vi "GSP_Manager_CF.vi"() -> ()   [LabVIEW 2015]
uses:
  SystemUtil/ScriptArray.ctl
  SystemUtil/Script.ctl
  SystemUtil/Command.ctl
  SystemUtil/MotorStates.ctl
  piezo_setpoint.ctl
  SystemUtil/ThreadStates.ctl
  Log/LogItem.ctl
  GSP_CF_Global.vi
  GUI/GSP_GUI_global.vi
panel:
  in  "Change CF":bool
  in  "CF Target":i32 caption="Target" min=-3000 max=3000
  out "CF Actual":i32 caption="Actual"
  out "Cameral Ext Temp":dbl(slide) scale=0.0..20.0
  out "Last Error":errorcluster
  in  "CommandQ":string
  # "Camera Focus"
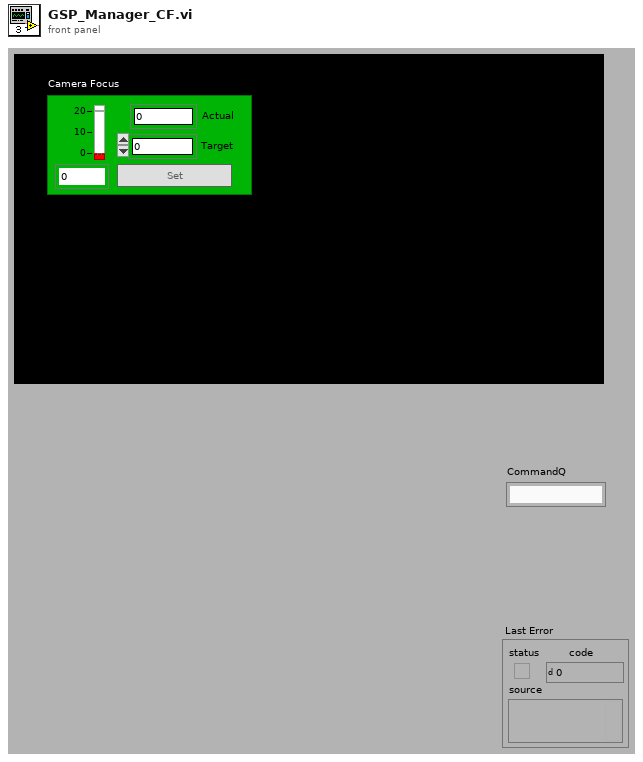
[diagram p1: front panel]
types:
  T1 = typedef "Command.ctl" = cluster{"Command":string, "Parameter":string}
  T2 = typedef "ScriptArray.ctl" = T3[]
  T3 = typedef "Script.ctl" = cluster{"Current Step":i32, "Commands":cluster{"Command":string, "Parameters":string}[]}
  T4 = cluster{"Move Mem Address":i32, "Home Mem Address":i32, "Adjust Piezo Address":i32}
  T5 = typedef "MotorStates.ctl" = enum16{"Ready", "Moving", "Uninitialized", "Error"}
  T6 = typedef "piezo_setpoint.ctl" = cluster{"Left":i32, "Right":i32}
  T7 = typedef "ThreadStates.ctl" = enum16{"Waiting", "Scripting", "Uninitialized", "Error"}
  T8 = enum16{"Launch", "Log", "Open", "Close", "Shutdown"}
  T9 = typedef "LogItem.ctl" = cluster{"error in (no error)":errorcluster, "Source":string, "Comment ":string}
  T10 = enum16{"POL (0)", "CPL (1)", "HLT (2)", "STP (3)", "RST (4)", "RVN (5)", "RPB (6)", "CLP (8)", "SDL (9)", "RUN (10)", "WRI (11)", "RRG (12)", "SPR (13)", "LPR (14)", "VMI (15)", "SSP (17)", "SSE (18)", "RIS (20)", "RIO (21)", "IMW (25)", "END (128)", "MAV (134)", "MRV (135)", "JRE (137)", "WCL (138)", "WCW (139)", "DLY (140)", "WDL (141)", "GCL (142)", "GOP (143)", "ZTG (144)", "ZTP (145)", "TTP (146)", "CME (147)", "CTC (148)", "TQL (149)", "AHC (150)", "ERL (151)", "OLP (152)", "WRP (154)", "IDT (155)", "LRP (156)", "VMP (159)", "RAV (160)", "RRV (161)", "JMP (162)", "JOI (162)", "CIS (163)", "CKS (164)", "CLC (165)", "KMC (167)", "MCT (168)", "FLC (169)", "EEM (170)", "DDB (171)", "DEM (171)", "PAC (172)", "ADL (173)", "BRT (174)", "MAT (176)", "MRT (177)", "RAT (178)", "RRT (179)", "SSD (180)", "KMR (181)", "KED (182)", "KDD (183)", "DIR (184)", "PRO (185)", "SIF (186)", "EDL (187)", "CIO (188)", "MDS (189)", "MDC (190)", "MDT (191)", "SEE (192)", "ARI (193)", "WBS (194)", "SCF (195)", "RSM (196)", "RLM (197)", "RSN (198)", "RLN (199)", "PCL (201)", "PCI (201)", "PRT (202)", "PRI (202)", "WBE (204)", "SOB (205)", "COB (206)", "ACR (207)", "PLR (208)", "CAI (211)", "LVT (212)", "OVT (213)", "MTT (214)", "CLC (215)", "PIM (216)", "VIM (217)", "TIM (218)", "AHM (219)", "SSL (221)", "TRU (222)", "RSD (223)", "EMT (225)", "DMT (226)", "EMD (227)", "DMD (228)", "HSM (229)", "AHD (230)", "PCM (231)", "PCG (232)", "XRV (233)", "XAV (234)", "XRT (235)", "XAT (236)", "GOC (237)", "JNA (238)", "JOR (239)", "PMC (240)", "PMV (241)", "PMX (242)", "DLC (243)", "SLC (244)", "PCP (245)", "ATR (248)", "PMO (249)", "JAN (250)", "EDH (251)", "DIF (252)", "IMS (253)", "IMQ (254)"}
  T11 = cluster{"Mount Az":dbl, "Mount El":dbl, "RA":string, "DEC":string, "Hour Angle":string, "Airmass":dbl, "Focus":dbl, "Rotator Angle":dbl, "Rotator Location":string, "Dome Shutter":string, "Dome Az":dbl, "Date":string, "UT Time":string, "Sidereal Time":string, "Position Angle":dbl, "Seeing":dbl, "OBSRA":string, "OBSDEC":string, "Position ADC":string, "Position ADC 2":string}
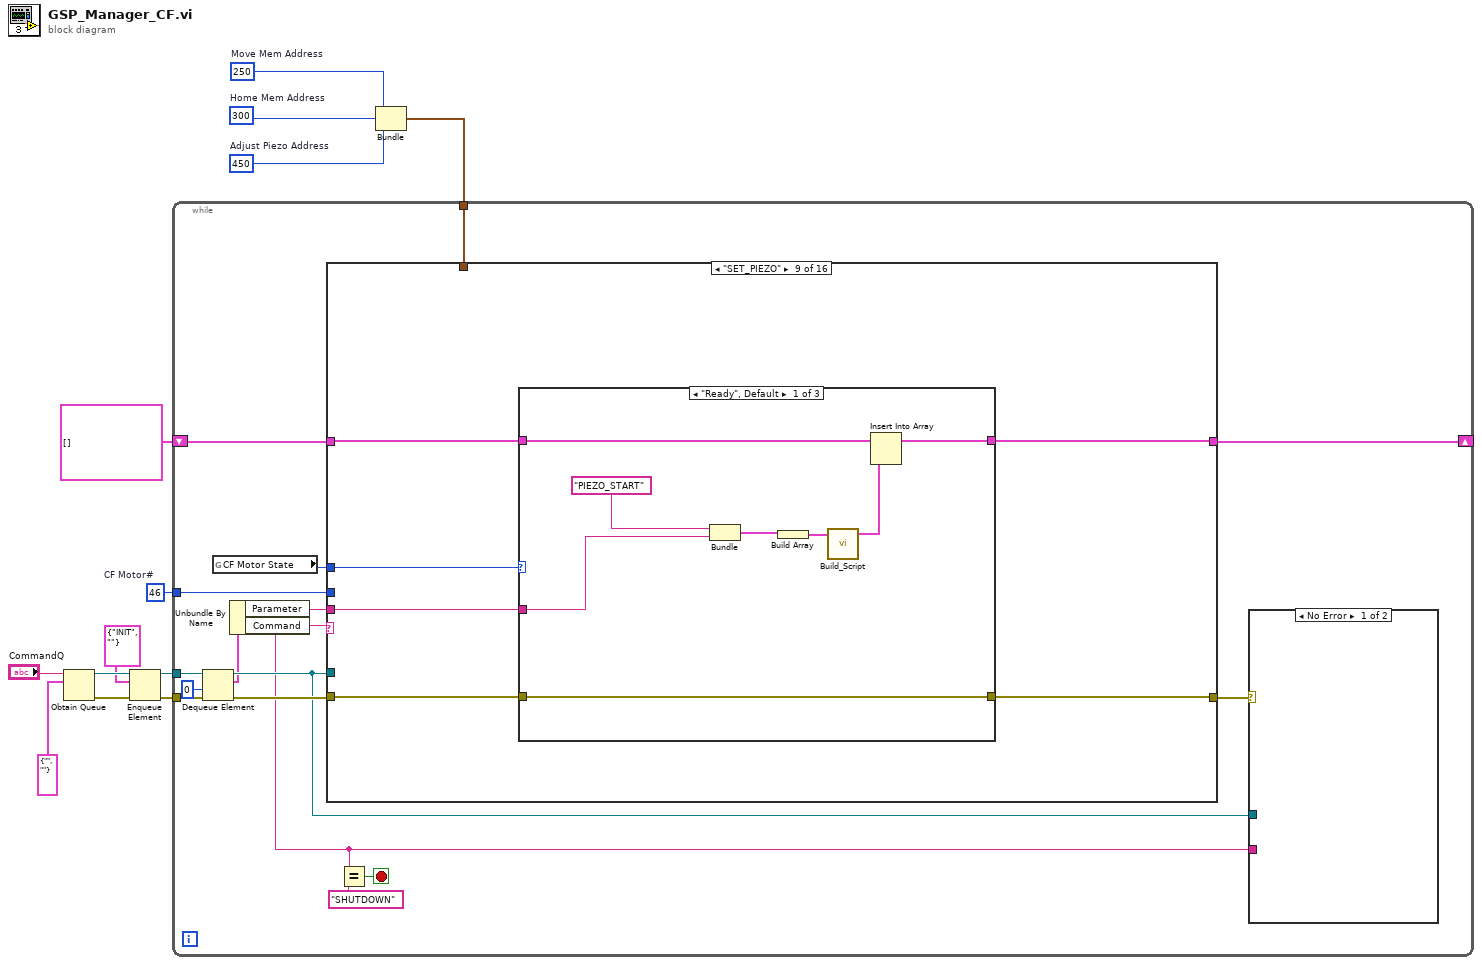
[diagram p0: block diagram]
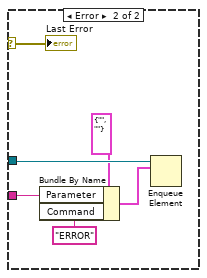
[diagram p2: hidden frame]
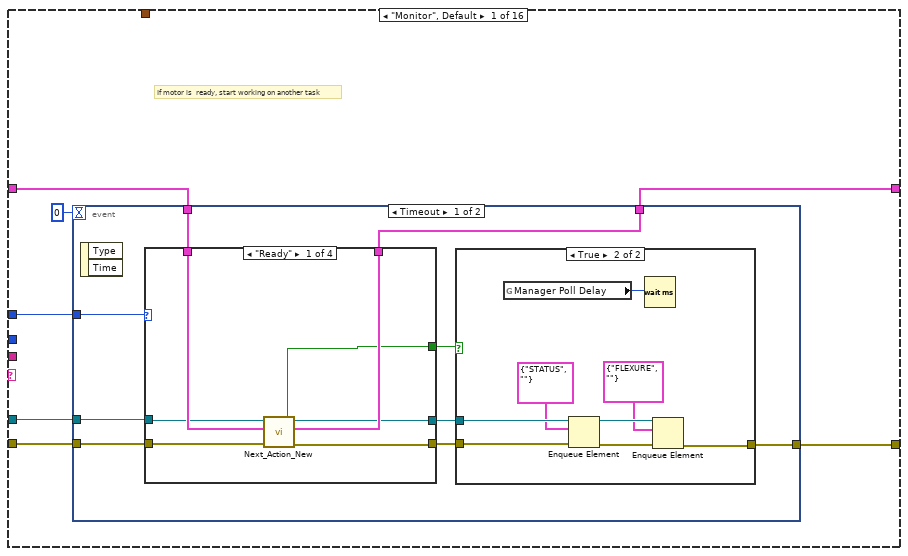
[diagram p3: hidden frame]
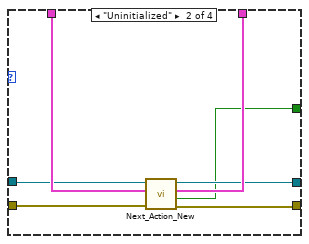
[diagram p5: hidden frame]
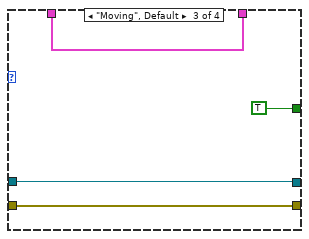
[diagram p6: hidden frame]
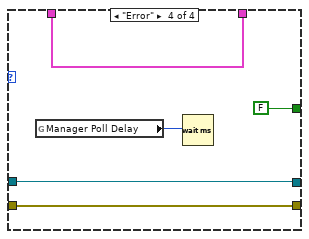
[diagram p7: hidden frame]
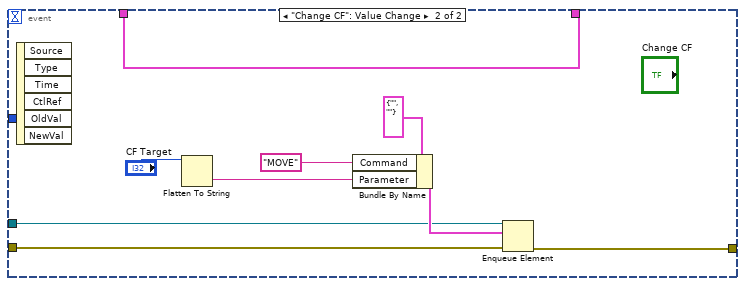
[diagram p8: hidden frame]
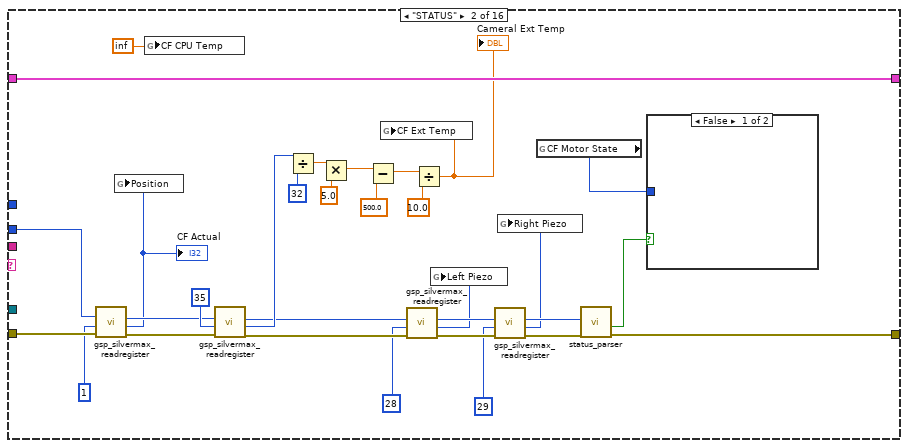
[diagram p9: hidden frame]
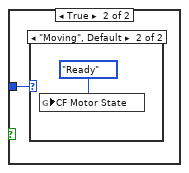
[diagram p10: hidden frame]
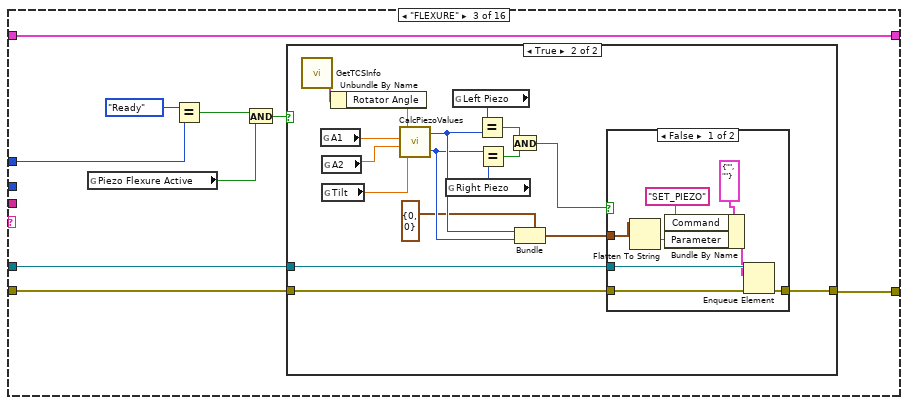
[diagram p12: hidden frame]
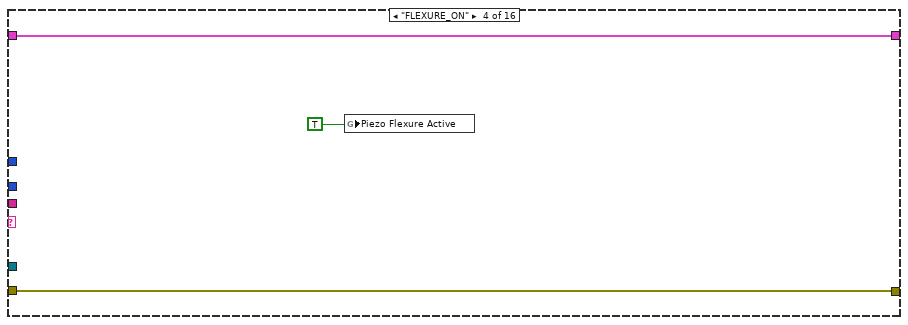
[diagram p15: hidden frame]
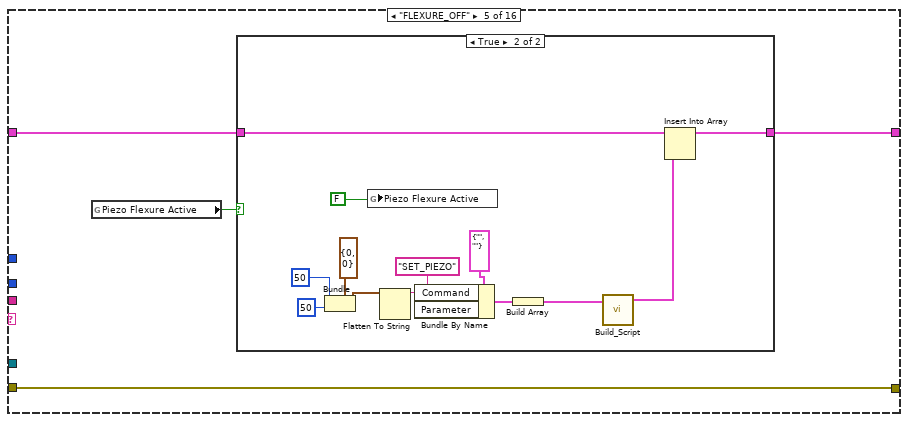
[diagram p16: hidden frame]
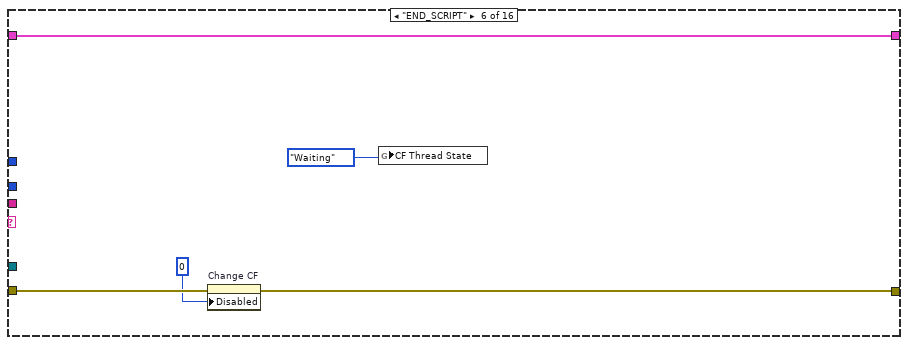
[diagram p18: hidden frame]
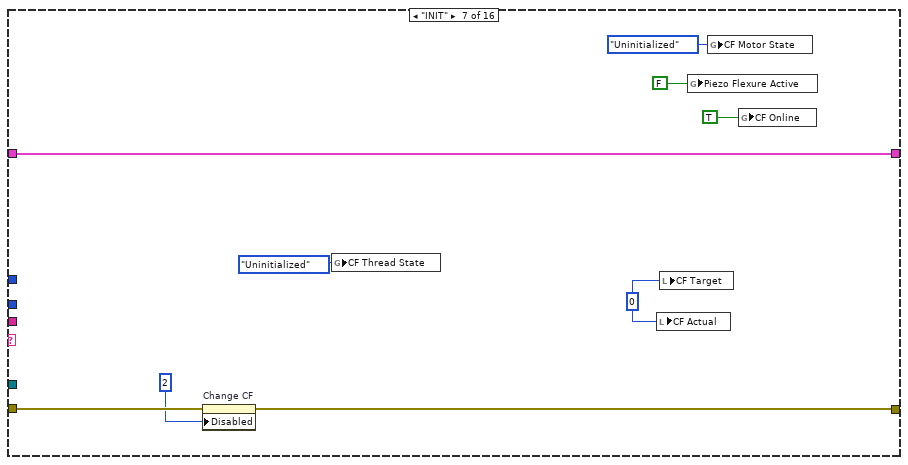
[diagram p19: hidden frame]
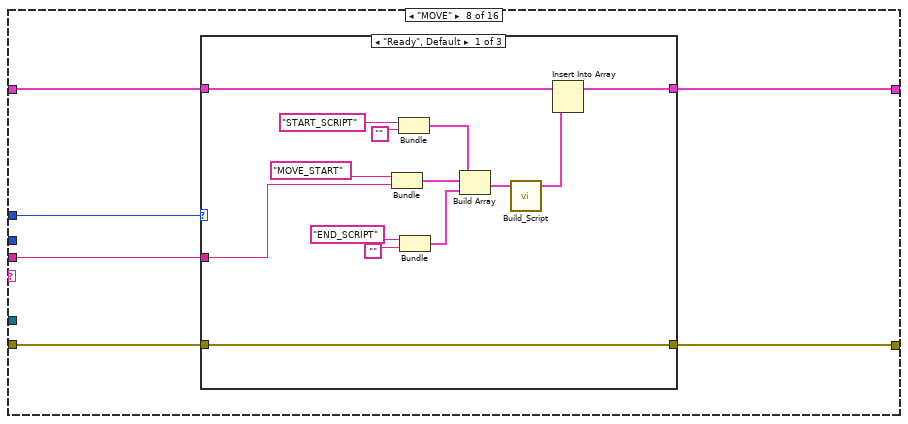
[diagram p20: hidden frame]
diagram:
  w1 = 450  # Adjust Piezo Address
  w3 = 300  # Home Mem Address
  w4 = 250  # Move Mem Address
  w5 = u8 46  # CF Motor#
  n1 = Obtain Queue(name (unnamed)="CommandQ", element data type=T1 {"Command"="", "Parameter"=""} ("Command")) -> (queue out=w10:refnum<queue>, error out=w11:errorcluster)  [unwired: 3 in, 1 out]
  n2 = Enqueue Element(queue=w10, element=T1 {"Command"="INIT", "Parameter"=""}, error in (no error)=w11) -> (queue out=w13:refnum<queue>, error out=w12:errorcluster)  [unwired: 1 in, 1 out]
  n3 = Bundle("Move Mem Address"=w4, "Home Mem Address"=w3, "Adjust Piezo Address"=w1) -> (w2:T4)  [unwired: 1 in]
  n4 = while {
    tunnel: w13 -> [w29]
    tunnel: w12 -> [w28]
    tunnel: w5 -> [w23]
    shift-right: [w22] -> _
    shift-left: T2 [] ("Operations") -> [w21]
    tunnel: w2 -> [w14]
    stop <- w17 stop-if-true
    n5 = Dequeue Element(queue=w29, timeout in ms (-1)=0, error in (no error)=w28) -> (queue out=w25:refnum<queue>, element=w19:T1, error out=w27:errorcluster)  [unwired: 1 out]
    n6 = global read "GSP_CF_Global.vi" "CF Motor State"() -> (w15:T5)
    n7 = Unbundle By Name(w19) -> ("Parameter"=w18:string, "Command"=w16:string)
    n8 = case shown="\"SET_PIEZO\"" w16 {
      tunnel: w27 -> [w41 w123 w131 w162 w166 w184 w189 w199 w235 w263 w282 w310 w316 w321 w324 _]
      tunnel: w25 -> [w42 _ w130 _ _ _ _ _ _ _ _ w311 _ _ _ w344]
      tunnel: [w37 w120 w129 w162 w166 w185 w190 w198 w234 w273 w298 w309 w314 w321 w330 _] -> w26
      tunnel: w23 -> [_ w122 _ _ _ _ _ _ _ w267 w290 _ _ _ w333 _]
      tunnel: w21 -> [w40 w118 w134 w164 w168 w187 w195 w202 w238 w270 w295 w312 w318 w323 w327 w338]
      tunnel: [w39 w118 w134 w164 w167 w187 w195 w201 w237 w270 w295 w312 w318 w322 w327 w337] -> w22
      tunnel: w18 -> [_ _ _ _ _ _ _ w200 w236 w268 w294 _ _ _ _ _]
      tunnel: w15 -> [w38 _ w127 _ _ _ _ w197 w233 _ _ _ _ _ _ _]
      tunnel: w14 -> [_ _ _ _ _ _ _ _ _ w266 w284 _ _ _ w326 _]
      frame "Monitor", Default {
        # "If motor is  ready, start working on another task"
        n9 = event shown="[0] Timeout" {
          selector: _ -> [_ _]
          dyn-events: _ -> [_ _]
          timeout: 0 -> [_ _]
          tunnel: w42 -> [w51 w88]
          tunnel: w41 -> [w50 w87]
          tunnel: w40 -> [w49 w84]
          tunnel: [w48 w84] -> w39
          tunnel: w38 -> [w47 _]
          tunnel: [w43 w86] -> w37
          event Timeout {
            n10 = event-data() -> ()  [unwired: 1 in, 2 out]
            n11 = case shown="\"Ready\"" w47 {
              tunnel: w51 -> [w63 w70 w77 w80]
              tunnel: w50 -> [w67 w74 w76 w82]
              tunnel: [w65 w72 w76 w82] -> w46
              tunnel: w49 -> [w66 w73 w78 w83]
              tunnel: [w64 w71 w78 w83] -> w48
              tunnel: [w62 w68 TRUE FALSE] -> w45
              tunnel: [w61 w69 w77 w80] -> w44
              frame "Ready" {
                n12 = call "Next_Action_New.vi"("error in (no error)"=w67, "Operations"=w66, "queue in"=w63) -> ("error out"=w65:errorcluster, "No command?"=w62:bool, "Operations Out"=w64:T2, "queue out"=w61:refnum<queue>)  [unwired: 1 in]
              }
              frame "Uninitialized" {
                n13 = call "Next_Action_New.vi"("error in (no error)"=w74, "Operations"=w73, "queue in"=w70) -> ("error out"=w72:errorcluster, "No command?"=w68:bool, "Operations Out"=w71:T2, "queue out"=w69:refnum<queue>)  [unwired: 1 in]
              }
              frame "Moving", Default {
              }
              frame "Error" {
                n14 = global read "GSP_GUI_global.vi" "Manager Poll Delay"() -> (w81:u32)
                n15 = Wait (ms)(milliseconds to wait=w81) -> ()  [unwired: 1 out]
              }
            }
            n16 = case shown="True" w45 {
              tunnel: w46 -> [w52 w60]
              tunnel: w44 -> [_ w59]
              tunnel: [w52 w53] -> w43
              frame False {
              }
              frame True {
                n17 = global read "GSP_GUI_global.vi" "Manager Poll Delay"() -> (w58:u32)
                n18 = Enqueue Element(queue=w59, element=T1 {"Command"="STATUS", "Parameter"=""}, error in (no error)=w60) -> (queue out=w57:refnum<queue>, error out=w56:errorcluster)  [unwired: 1 in, 1 out]
                n19 = Wait (ms)(milliseconds to wait=w58) -> ()  [unwired: 1 out]
                n20 = Enqueue Element(queue=w57, element=cluster{"Command":string, "Parameters":string} {"Command"="FLEXURE", "Parameters"=""} ("Default Command"), error in (no error)=w56) -> (error out=w53:errorcluster)  [unwired: 1 in, 2 out]
              }
            }
          }
          event "Change CF": Value Change {
            n21 = event-data() -> ()  [unwired: 1 in, 6 out]
            n22 = Flatten To String(anything="CF Target") -> (data string=w89:string)  [unwired: 3 in, 2 out]
            n23 = Bundle By Name(cluster=T1 {"Command"="", "Parameter"=""} ("element"), "Command"="MOVE" ("element"), "Parameter"=w89) -> (w91:T1)
            n24 = Enqueue Element(queue=w88, element=w91, error in (no error)=w87) -> (error out=w86:errorcluster)  [unwired: 1 in, 2 out]
          }
        }
      }
      frame "STATUS" {
        n25 = call "gsp_silvermax_readregister.vi"("error in (no error)"=w123, "Register# (0)"=u8 1, "Motor #"=w122) -> ("error out"=w115:errorcluster, "Register Value"=w93:i32, "Motor # dup"=w116:u8)  [unwired: 2 in, 2 out]
        "CF Actual" <- w93
        n26 = global write "GSP_CF_Global.vi" "Position"(w93) -> ()
        n27 = global write "GSP_CF_Global.vi" "CF CPU Temp"(inf) -> ()
        n28 = call "gsp_silvermax_readregister.vi"("error in (no error)"=w115, "Register# (0)"=u8 35, "Motor #"=w116) -> ("error out"=w105:errorcluster, "Register Value"=w106:i32, "Motor # dup"=w104:u8)  [unwired: 2 in, 2 out]
        n29 = Divide(x=w106, y=32) -> (x/y=w113:dbl)
        n30 = Multiply(x=w113, y=5.0) -> (x*y=w111:dbl)
        n31 = Subtract(x=w111, y=500.0) -> (x-y=w109:dbl)
        n32 = call "gsp_silvermax_readregister.vi"("error in (no error)"=w105, "Register# (0)"=u8 28, "Motor #"=w104) -> ("error out"=w102:errorcluster, "Register Value"=w97:i32, "Motor # dup"=w100:u8)  [unwired: 2 in, 2 out]
        n33 = Divide(x=w109, y=10.0) -> (x/y=w94:dbl)
        "Cameral Ext Temp" <- w94
        n34 = global write "GSP_CF_Global.vi" "CF Ext Temp"(w94) -> ()
        n35 = global write "GSP_CF_Global.vi" "Left Piezo"(w97) -> ()
        n36 = call "gsp_silvermax_readregister.vi"("error in (no error)"=w102, "Register# (0)"=u8 29, "Motor #"=w100) -> ("error out"=w101:errorcluster, "Register Value"=w96:i32, "Motor # dup"=w99:u8)  [unwired: 2 in, 2 out]
        n37 = global write "GSP_CF_Global.vi" "Right Piezo"(w96) -> ()
        n38 = global read "GSP_CF_Global.vi" "CF Motor State"() -> (w95:T5)
        n39 = call "status_parser.vi"("error in (no error)"=w101, "Motor #"=w99) -> ("error out"=w120:errorcluster, "Program Complete?"=w119:bool)  [unwired: 3 in, 1 out]
        n40 = case shown="False" w119 {
          tunnel: w95 -> [_ w124]
          frame False {
          }
          frame True {
            n41 = case shown="\"Moving\", Default" w124 {
              frame "Uninitialized" {
              }
              frame "Moving", Default {
                n42 = global write "GSP_CF_Global.vi" "CF Motor State"(MotorStates."Ready" ("Mode")) -> ()
              }
            }
          }
        }
      }
      frame "FLEXURE" {
        n43 = global read "GSP_CF_Global.vi" "Piezo Flexure Active"() -> (w128:bool)
        n44 = Equal?(x=MotorStates."Ready", y=w127) -> (x = y?=w133:bool)
        n45 = And(x=w133, y=w128) -> (x .and. y?=w132:bool)
        n46 = case shown="True" w132 {
          tunnel: w131 -> [w135 w143]
          tunnel: w130 -> [_ w144]
          tunnel: [w135 w145] -> w129
          frame False {
          }
          frame True {
            n47 = call "GetTCSInfo.vi"() -> ("TCSInfo"=w137:T11)
            n48 = global read "GSP_CF_Global.vi" "A1"() -> (w152:dbl)
            n49 = global read "GSP_CF_Global.vi" "A2"() -> (w151:dbl)
            n50 = global read "GSP_CF_Global.vi" "Tilt"() -> (w150:dbl)
            n51 = Unbundle By Name(w137) -> ("Rotator Angle"=w136:dbl)
            n52 = call "CalcPiezoValues.vi"("Tilt"=w150, "A2"=w151, "A1"=w152, "Rotator Position"=w136) -> ("Right Piezo"=w141:i32, "Left Piezo"=w142:i32)
            n53 = global read "GSP_CF_Global.vi" "Right Piezo"() -> (w148:i32)
            n54 = global read "GSP_CF_Global.vi" "Left Piezo"() -> (w149:i32)
            n55 = Equal?(x=w149, y=w142) -> (x = y?=w147:bool)
            n56 = Equal?(x=w141, y=w148) -> (x = y?=w146:bool)
            n57 = And(x=w147, y=w146) -> (x .and. y?=w140:bool)
            n58 = Bundle(cluster=T6 {"Left"=0, "Right"=0} ("Piezos Setpoints"), "Left"=w142, "Right"=w141) -> (w139:T6)
            n59 = case shown="False" w140 {
              tunnel: [w160 w161] -> w145
              tunnel: w144 -> [w159 _]
              tunnel: w143 -> [w158 w161]
              tunnel: w139 -> [w154 _]
              frame False {
                n60 = Flatten To String(anything=w154) -> (data string=w153:string)  [unwired: 3 in, 2 out]
                n61 = Bundle By Name(cluster=T1 {"Command"="", "Parameter"=""} ("element"), "Command"="SET_PIEZO", "Parameter"=w153) -> (w155:T1)
                n62 = Enqueue Element(queue=w159, element=w155, error in (no error)=w158) -> (error out=w160:errorcluster)  [unwired: 1 in, 2 out]
              }
              frame True {
              }
            }
          }
        }
      }
      frame "FLEXURE_ON" {
        n63 = global write "GSP_CF_Global.vi" "Piezo Flexure Active"(TRUE) -> ()
      }
      frame "FLEXURE_OFF" {
        n64 = global read "GSP_CF_Global.vi" "Piezo Flexure Active"() -> (w165:bool)
        n65 = case shown="True" w165 {
          tunnel: w168 -> [w169 w174]
          tunnel: [w169 w170] -> w167
          frame False {
          }
          frame True {
            n66 = Bundle(cluster=T6 {"Left"=0, "Right"=0} ("Piezos Setpoints"), "Left"=50, "Right"=50) -> (w177:T6)
            n67 = global write "GSP_CF_Global.vi" "Piezo Flexure Active"(FALSE) -> ()
            n68 = Flatten To String(anything=w177) -> (data string=w179:string)  [unwired: 3 in, 2 out]
            n69 = Bundle By Name(cluster=T1 {"Command"="", "Parameter"=""} ("element"), "Command"="SET_PIEZO", "Parameter"=w179) -> (w172:T1)
            n70 = Build Array(w172) -> (w171:T1[])
            n71 = call "Build_Script.vi"("Commands"=w171) -> ("script out"=w173:T3)  [unwired: 4 in]
            n72 = Insert Into Array(array=w174, new element=w173) -> (w170:T2)  [unwired: 1 in]
          }
        }
      }
      frame "END_SCRIPT" {
        n73 = property on="Change CF" class="Bool"(error in=w184, "Disabled"=u8 0) -> (error out=w185:errorcluster)  [unwired: 1 in, 1 out]
        n74 = global write "GSP_CF_Global.vi" "CF Thread State"(ThreadStates."Waiting" ("Thread state")) -> ()
      }
      frame "INIT" {
        w191 = 0 ("Value")
        n75 = property on="Change CF" class="Bool"(error in=w189, "Disabled"=u8 2) -> (error out=w190:errorcluster)  [unwired: 1 in, 1 out]
        n76 = global write "GSP_CF_Global.vi" "CF Thread State"(ThreadStates."Uninitialized" ("Thread state")) -> ()
        n77 = local write "CF Actual"(w191) -> ()
        n78 = local write "CF Target"(w191) -> ()
        n79 = global write "GSP_CF_Global.vi" "Piezo Flexure Active"(FALSE) -> ()
        n80 = global write "GSP_CF_Global.vi" "CF Motor State"(MotorStates."Uninitialized" ("Mode")) -> ()
        n81 = global write "GSP_CF_Global.vi" "CF Online"(TRUE ("CS Online")) -> ()
      }
      frame "MOVE" {
        n82 = case shown="\"Ready\", Default" w197 {
          tunnel: w202 -> [w216 w218 w226]
          tunnel: [w215 w218 w226] -> w201
          tunnel: w200 -> [w209 _ _]
          tunnel: w199 -> [w214 w224 w232]
          tunnel: [w214 w223 w231] -> w198
          frame "Ready", Default {
            n83 = Bundle("MOVE_START", "Parameter"=w209) -> (w208:cluster{string, "Parameter":string})  [unwired: 1 in]
            n84 = Bundle("START_SCRIPT", "") -> (w203:cluster{string, string})  [unwired: 1 in]
            n85 = Bundle("END_SCRIPT", "") -> (w207:cluster{string, string})  [unwired: 1 in]
            n86 = Build Array(w203, w208, w207) -> (w206:cluster{string, "Parameter":string}[])
            n87 = call "Build_Script.vi"("Commands"=w206) -> ("script out"=w213:T3)  [unwired: 4 in]
            n88 = Insert Into Array(array=w216, new element=w213) -> (w215:T2)  [unwired: 1 in]
          }
          frame "Uninitialized" {
            n89 = Bundle By Name(cluster=T9 {"error in (no error)"={"status"=FALSE, "code"=0, "source"=""}, "Source"="", "Comment "=""} ("Log"), "Source"="Coll Focus Manager", "Comment"="Cannot perform move") -> (w222:T9)
            n90 = call "GSP_Logger_Handler.vi"("error in (no error)"=w224, "Log"=w222, "Actions"=T8."Log") -> ("error out"=w223:errorcluster)  [unwired: 4 in]
          }
          frame "Error" {
            n91 = Bundle By Name(cluster=T9 {"error in (no error)"={"status"=FALSE, "code"=0, "source"=""}, "Source"="", "Comment "=""} ("Log"), "Source"="Coll Focus Manager", "Comment"="Cannot perform move") -> (w230:T9)
            n92 = call "GSP_Logger_Handler.vi"("error in (no error)"=w232, "Log"=w230, "Actions"=T8."Log") -> ("error out"=w231:errorcluster)  [unwired: 4 in]
          }
        }
      }
      frame "SET_PIEZO" {
        n93 = case shown="\"Ready\", Default" w233 {
          tunnel: w238 -> [w246 w248 w256]
          tunnel: [w245 w248 w256] -> w237
          tunnel: w236 -> [w241 _ _]
          tunnel: w235 -> [w244 w254 w262]
          tunnel: [w244 w253 w261] -> w234
          frame "Ready", Default {
            n94 = Bundle("PIEZO_START", "Parameter"=w241) -> (w240:cluster{string, "Parameter":string})  [unwired: 1 in]
            n95 = Build Array(w240) -> (w239:cluster{string, "Parameter":string}[])
            n96 = call "Build_Script.vi"("Commands"=w239) -> ("script out"=w243:T3)  [unwired: 4 in]
            n97 = Insert Into Array(array=w246, new element=w243) -> (w245:T2)  [unwired: 1 in]
          }
          frame "Uninitialized" {
            n98 = Bundle By Name(cluster=T9 {"error in (no error)"={"status"=FALSE, "code"=0, "source"=""}, "Source"="", "Comment "=""} ("Log"), "Source"="Camera Focus Manager", "Comment"="Cannot perform move") -> (w252:T9)
            n99 = call "GSP_Logger_Handler.vi"("error in (no error)"=w254, "Log"=w252, "Actions"=T8."Log") -> ("error out"=w253:errorcluster)  [unwired: 4 in]
          }
          frame "Error" {
            n100 = Bundle By Name(cluster=T9 {"error in (no error)"={"status"=FALSE, "code"=0, "source"=""}, "Source"="", "Comment "=""} ("Log"), "Source"="Camera Focus Manager", "Comment"="Cannot perform move") -> (w260:T9)
            n101 = call "GSP_Logger_Handler.vi"("error in (no error)"=w262, "Log"=w260, "Actions"=T8."Log") -> ("error out"=w261:errorcluster)  [unwired: 4 in]
          }
        }
      }
      frame "MOVE_START" {
        n102 = Unflatten From String(type=0, binary string=w268) -> (value=w264:i32)  [unwired: 3 in, 2 out]
        n103 = Unbundle By Name(w266) -> ("Move Mem Address"=w265:i32)
        n104 = local write "CF Target"(w264) -> ()
        n105 = global write "GSP_CF_Global.vi" "Target"(w264) -> ()
        n106 = Number To Decimal String(number=w265) -> (decimal integer string=w272:string)  [unwired: 1 in]
        n107 = call "gsp_silvermax_writeregister.vi"("error in (no error)"=w263, "Register Value"=w264, "Motor #"=w267, "Register# (0)"=u8 25) -> ("error out"=w277:errorcluster, "Motor # dup"=w275:u8)  [unwired: 2 in]
        n108 = Build Array(w272) -> (w271:string[])
        n109 = call "gsp_silvermax_commandreponse.vi"("error in (no error)"=w277, "Parameters (none)"=w271, "Motor #"=w275, "Command"=T10."LRP (156)") -> ("error out"=w274:errorcluster)  [unwired: 3 out]
        n110 = case shown="No Error" w274 {
          selector: w274 -> [w280 w281]
          tunnel: [w280 w281] -> w273
          frame No Error {
            n111 = global write "GSP_CF_Global.vi" "CF Motor State"(MotorStates."Moving" ("Mode")) -> ()
          }
          frame Error {
          }
        }
      }
      frame "PIEZO_START" {
        n112 = Unflatten From String(type=T6 {"Left"=0, "Right"=0} ("Piezos Setpoints"), binary string=w294) -> (value=w291:T6)  [unwired: 3 in, 2 out]
        n113 = Unbundle By Name(w291) -> ("Left"=w288:i32, "Right"=w287:i32)
        n114 = Unbundle By Name(w284) -> ("Adjust Piezo Address"=w283:i32)
        n115 = call "gsp_silvermax_writeregister.vi"("error in (no error)"=w282, "Register Value"=w288, "Motor #"=w290, "Register# (0)"=u8 30) -> ("error out"=w293:errorcluster, "Motor # dup"=w289:u8)  [unwired: 2 in]
        n116 = Number To Decimal String(number=w283) -> (decimal integer string=w297:string)  [unwired: 1 in]
        n117 = call "gsp_silvermax_writeregister.vi"("error in (no error)"=w293, "Register Value"=w287, "Motor #"=w289, "Register# (0)"=u8 31) -> ("error out"=w302:errorcluster, "Motor # dup"=w300:u8)  [unwired: 2 in]
        n118 = Build Array(w297) -> (w296:string[])
        n119 = call "gsp_silvermax_commandreponse.vi"("error in (no error)"=w302, "Parameters (none)"=w296, "Motor #"=w300, "Command"=T10."LRP (156)") -> ("error out"=w299:errorcluster)  [unwired: 3 out]
        n120 = case shown="No Error" w299 {
          selector: w299 -> [w304 w305]
          tunnel: [w304 w305] -> w298
          frame No Error {
            n121 = global write "GSP_CF_Global.vi" "CF Motor State"(MotorStates."Moving" ("Mode")) -> ()
          }
          frame Error {
          }
        }
      }
      frame "SHUTDOWN" {
        n122 = Release Queue(queue=w311, error in (no error)=w310) -> (error out=w306:errorcluster)  [unwired: 1 in, 2 out]
        n123 = global write "GSP_CF_Global.vi" "CF Thread State"(ThreadStates."Uninitialized" ("Thread state")) -> ()
        n124 = property on="Change CF" class="Bool"(error in=w306, "Disabled"=u8 2) -> (error out=w309:errorcluster)  [unwired: 1 in, 1 out]
        n125 = stacked-sequence {
          tunnel: w309 -> [_]
          frame #0 {
            n126 = global write "GSP_CF_Global.vi" "CF Online"(FALSE ("CS Online")) -> ()
          }
        }
      }
      frame "START_SCRIPT" {
        n127 = property on="Change CF" class="Bool"(error in=w316, "Disabled"=u8 2) -> (error out=w314:errorcluster)  [unwired: 1 in, 1 out]
        n128 = global write "GSP_CF_Global.vi" "CF Thread State"(ThreadStates."Scripting" ("Thread state")) -> ()
      }
      frame "HOME" {
        n129 = call "Build_Script.vi"("Commands"=cluster{"Command":string, "Parameters":string}[] [{"Command"="START_SCRIPT", "Parameters"=""}, {"Command"="HOME_START", "Parameters"=""}, {"Command"="END_SCRIPT", "Parameters"=""}]) -> ("script out"=w319:T3)  [unwired: 4 in]
        n130 = Insert Into Array(array=w323, new element=w319) -> (w322:T2)  [unwired: 1 in]
      }
      frame "HOME_START" {
        n131 = Unbundle By Name(w326) -> ("Home Mem Address"=w325:i32)
        n132 = Number To Decimal String(number=w325) -> (decimal integer string=w329:string)  [unwired: 1 in]
        n133 = Build Array(w329) -> (w328:string[])
        n134 = call "gsp_silvermax_commandreponse.vi"("error in (no error)"=w324, "Parameters (none)"=w328, "Motor #"=w333, "Command"=T10."LRP (156)") -> ("error out"=w331:errorcluster)  [unwired: 3 out]
        n135 = case shown="No Error" w331 {
          selector: w331 -> [w335 w336]
          tunnel: [w335 w336] -> w330
          frame No Error {
            n136 = global write "GSP_CF_Global.vi" "CF Motor State"(MotorStates."Moving" ("Mode")) -> ()
          }
          frame Error {
          }
        }
      }
      frame "ERROR" {
        n137 = local read "Last Error"() -> (w339:errorcluster)
        n138 = Unbundle By Name(w339) -> ("code"=w346:i32)
        n139 = Bundle By Name(cluster=T9 {"error in (no error)"={"status"=FALSE, "code"=0, "source"=""}, "Source"="", "Comment "=""} ("Log"), "error in (no error)"=w339, "Source"="CF Manager") -> (w341:T9)
        n140 = call "GSP_Logger_Handler.vi"("Log"=w341, "Actions"=T8."Log") -> ()  [unwired: 5 in, 1 out]
        n141 = case shown="0, Default" w346 {
          tunnel: w339 -> [_ _ _]
          tunnel: [errorcluster {"status"=FALSE, "code"=0, "source"=""} ("Last Error") errorcluster {"status"=FALSE, "code"=0, "source"=""} ("Last Error") errorcluster {"status"=FALSE, "code"=0, "source"=""} ("Last Error")] -> w345
          tunnel: w338 -> [_ w354 w356]
          tunnel: [T2 [] ("Operations") w354 w356] -> w337
          frame 0, Default {
            (unwired) u8 2 ("Disabled")
            n142 = global write "GSP_CF_Global.vi" "CF Motor State"(MotorStates."Error" ("Mode")) -> ()
            n143 = global write "GSP_CF_Global.vi" "CF Thread State"(ThreadStates."Error" ("Thread state")) -> ()
          }
          frame 5003, 5006 {
          }
          frame 5013 {
          }
        }
        n144 = case shown="No Error" w345 {
          tunnel: w344 -> [_ w348]
          frame No Error {
          }
          frame Error {
            n145 = Enqueue Element At Opposite End(queue=w348, element=T1 {"Command"="SHUTDOWN", "Parameter"=""}) -> ()  [unwired: 2 in, 3 out]
          }
        }
      }
    }
    n146 = Equal?(x=w16, y="SHUTDOWN") -> (x = y?=w17:bool)
    n147 = case shown="No Error" w26 {
      selector: w26 -> [_ w34]
      tunnel: w25 -> [_ w35]
      tunnel: w16 -> [_ w32]
      frame No Error {
      }
      frame Error {
        n148 = Bundle By Name(cluster=T1 {"Command"="", "Parameter"=""} ("element"), "Parameter"=w32, "Command"="ERROR" ("element")) -> (w30:T1)
        n149 = Enqueue Element(queue=w35, element=w30) -> ()  [unwired: 2 in, 3 out]
        "Last Error" <- w34
      }
    }
  }
